vi "sum of 3 Gaussians with offset model.vi"(3 "output control":T1, 4 "data":variant, 5 "X":dbl[](array[numeric]), 6 "a":dbl[](array[numeric])) -> (0 "error out":errorcluster, 1 "f'(X,a)":dbl[][](array[numeric]), 2 "f(X,a)":dbl[](array[numeric]))   [LabVIEW 2023]
doc: "Sum of three Gaussians, plus DC offset."
uses:
  <vilib>/gmath/NumericalOptimization/LM_output select.ctl
  <vilib>/gmath/NI_Gmath.lvlib
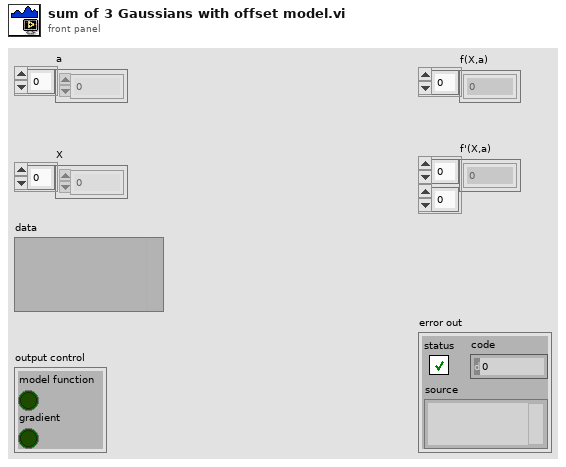
[diagram p1: front panel]
types:
  T1 = typedef "NI_Gmath.lvlib/LM_output select.ctl" = cluster{"model function":bool, "gradient":bool}
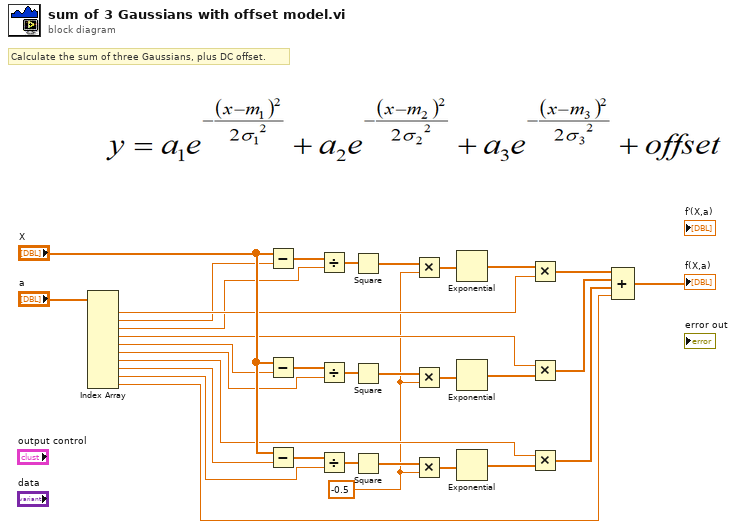
[diagram p0: block diagram]
diagram:
  w1 = -0.5
  # "Calculate the sum of three Gaussians, plus DC offset."
  n1 = Index Array(array="a") -> (element #1=w31:dbl, element #2=w30:dbl, element #3=w29:dbl, element #4=w28:dbl, element #5=w27:dbl, element #6=w26:dbl, element #7=w25:dbl, element #8=w24:dbl, element #9=w23:dbl, element #10=w22:dbl)  [unwired: 10 in]
  n2 = Subtract(x="X", y=w30) -> (x-y=w7:dbl[])
  n3 = Subtract(x="X", y=w27) -> (x-y=w5:dbl[])
  n4 = Subtract(x="X", y=w24) -> (x-y=w6:dbl[])
  n5 = Divide(x=w7, y=w29) -> (x/y=w19:dbl[])
  n6 = Divide(x=w5, y=w26) -> (x/y=w16:dbl[])
  n7 = Divide(x=w6, y=w23) -> (x/y=w15:dbl[])
  n8 = Square(x=w19) -> (x^2=w4:dbl[])
  n9 = Square(x=w16) -> (x^2=w3:dbl[])
  n10 = Square(x=w15) -> (x^2=w2:dbl[])
  n11 = Multiply(x=w4, y=w1) -> (x*y=w10:dbl[])
  n12 = Multiply(x=w3, y=w1) -> (x*y=w9:dbl[])
  n13 = Multiply(x=w2, y=w1) -> (x*y=w8:dbl[])
  n14 = Exponential(1:w10) -> (0:w18:dbl[])
  n15 = Exponential(1:w9) -> (0:w17:dbl[])
  n16 = Exponential(1:w8) -> (0:w14:dbl[])
  n17 = Multiply(x=w18, y=w31) -> (x*y=w13:dbl[])
  n18 = Multiply(x=w28, y=w17) -> (x*y=w12:dbl[])
  n19 = Multiply(x=w25, y=w14) -> (x*y=w11:dbl[])
  n20 = Compound Arithmetic op=ADD(w13, w12, w11, w22) -> (→"f(X,a)":dbl[])
